vi "WC Get Waveform Subset CDBL.vi"(4 "open interval? (T)":bool=TRUE, 5 "start/duration format":u16(ring) items=["Samples", "Relative Time"], 6 "error in (no error)":errorcluster, 7 "duration":dbl=1.0 format="%0.2f", 8 "start samples/time":dbl format="%0.2f", 9 "Waveform In":cluster{"t0":dbl, "dt":dbl, "Y":cdb[]} {"Y" format="%.3p"; "dt" format="%.6p"; "t0" format="%.6p"}) -> (0 "error out":errorcluster, 1 "actual duration":dbl format="%0.2f", 2 "actual start samples/time":dbl format="%0.2f", 3 "Waveform Out":cluster{"t0":dbl, "dt":dbl, "Y":cdb[]} {"Y" format="%.3p"; "dt" format="%.6p"; "t0" format="%.6p"})   [LabVIEW 2018]
doc: "Retrieves a subset of a waveform at a specified time or index. You must manually select the polymorphic instance you want to use."
panel:
  # "open"
  # "closed"
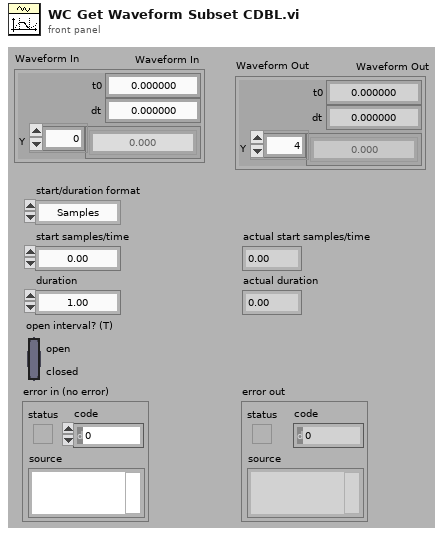
[diagram p1: front panel]
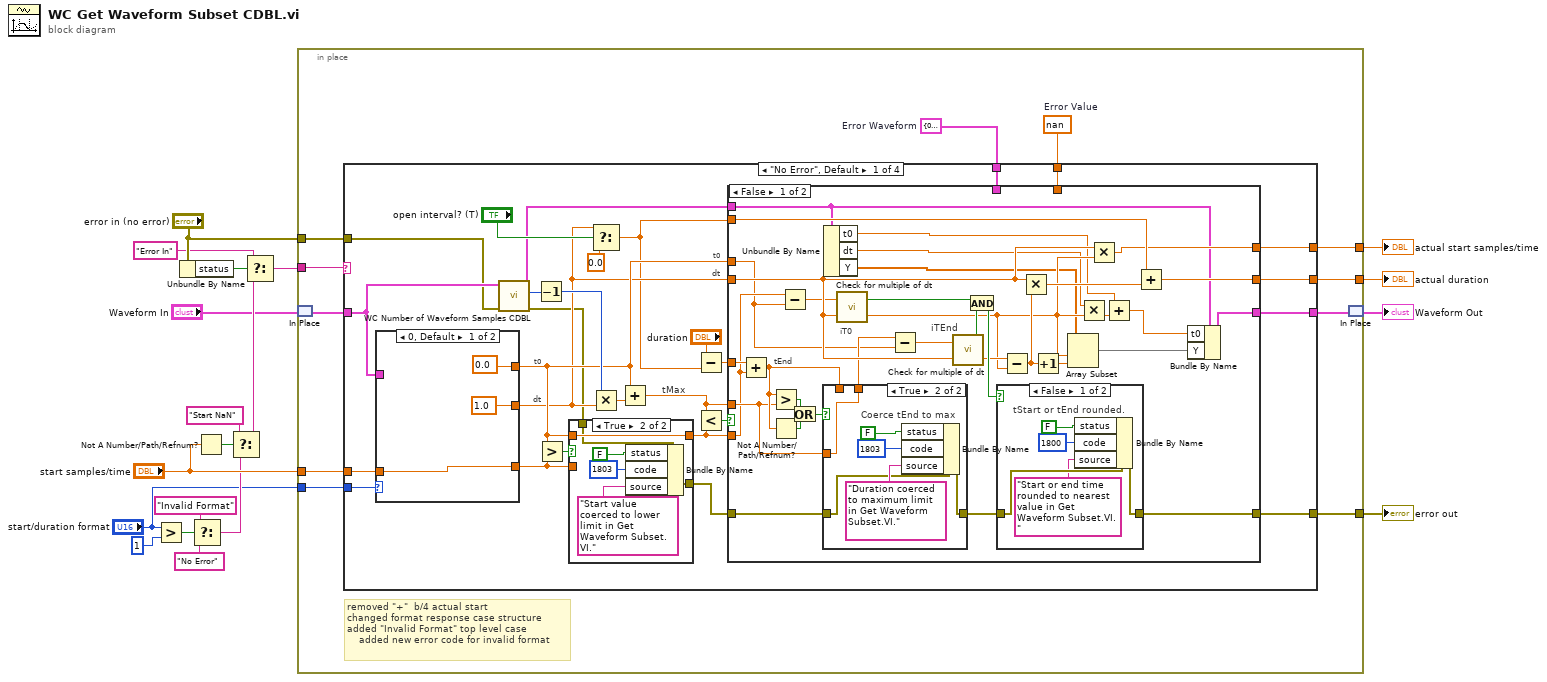
[diagram p0: block diagram]
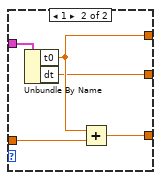
[diagram p2: hidden frame]
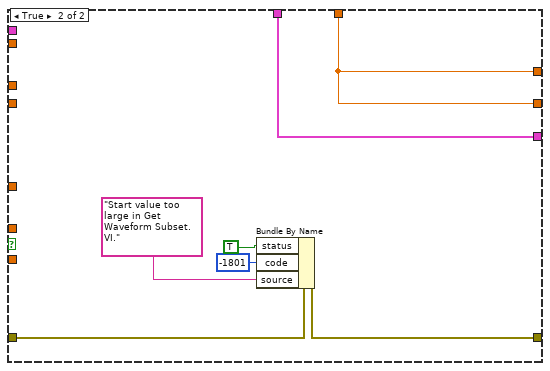
[diagram p5: hidden frame]
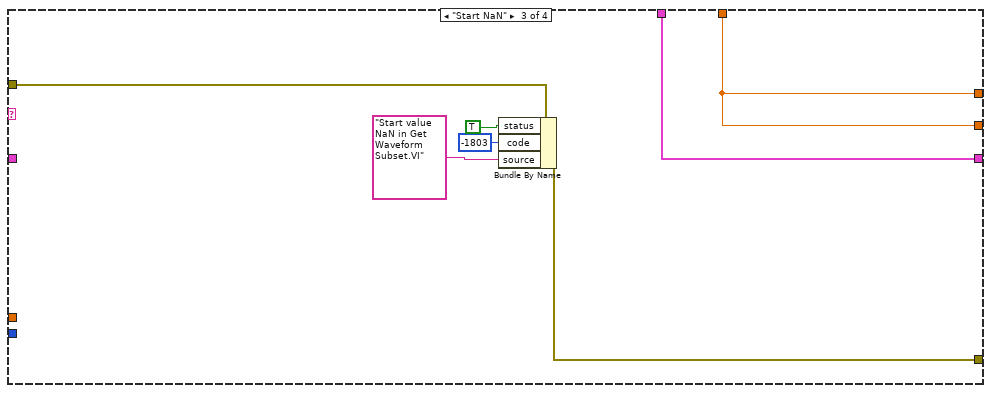
[diagram p8: hidden frame]
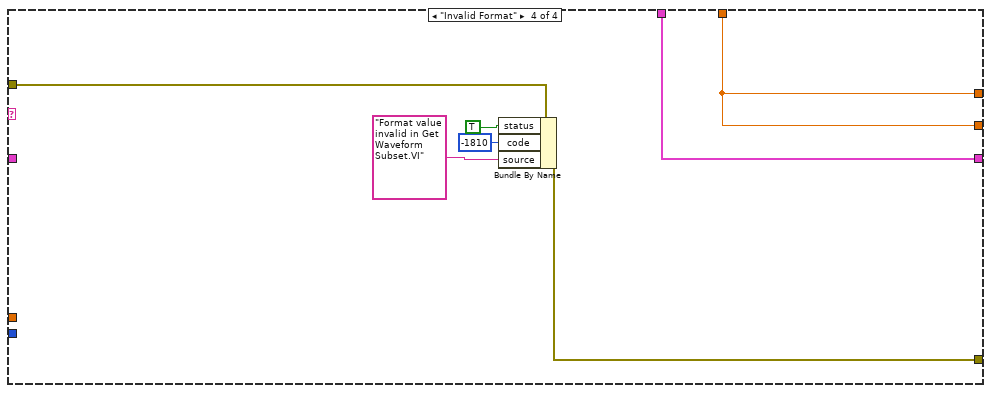
[diagram p9: hidden frame]
diagram:
  n1 = Greater?(x="start/duration format", y=u16 1) -> (0:w7:bool)
  n2 = Unbundle By Name("error in (no error)") -> ("status"=w17:bool)
  n3 = Select(t="Invalid Format", s=w7, f="No Error") -> (s? t:f=w5:string)
  n4 = Not A Number/Path/Refnum?(number/path/refnum="start samples/time") -> (NaN/Path/Refnum?=w19:bool)
  n5 = Select(t="Start NaN", s=w19, f=w5) -> (s? t:f=w15:string)
  n6 = Select(t="Error In", s=w17, f=w15) -> (s? t:f=w12:string)
  n7 = in-place {
    in-place-border: "error in (no error)" -> [w30]
    in-place-border: "start samples/time" -> [w29]
    in-place-border: w12 -> [w28]
    in-place-border: [w27] -> w11
    in-place-border: [w25] -> w10
    in-place-border: [w24] -> w9
    in-place-border: "start/duration format" -> [w23]
    w20 = cluster{"t0":dbl, "dt":dbl, "Y":cdb[]} {"t0"=0.0, "dt"=0.0, "Y"=[]}  # Error Waveform
    w26 = nan  # Error Value
    # "removed \"+\"  b/4 actual start\nchanged format response case structure\nadded \"Invalid Format\" top level case\n    added new error code for invalid format"
    n8 = in-place-match #1("Waveform In") -> (w22:cluster{"t0":dbl, "dt":dbl, "Y":cdb[]})
    n9 = case shown="\"No Error\", Default" w28 {
      tunnel: w22 -> [w33 _ _ _]
      tunnel: w30 -> [w31 w132 w139 w146]
      tunnel: w29 -> [w38 _ _ _]
      tunnel: [w48 w132 w138 w145] -> w27
      tunnel: [w50 w131 w134 w141] -> w21
      tunnel: w20 -> [w49 w131 w134 w141]
      tunnel: [w51 w130 w133 w140] -> w25
      tunnel: w26 -> [w52 w130 w133 w140]
      tunnel: [w47 w130 w133 w140] -> w24
      tunnel: w23 -> [w32 _ _ _]
      frame "No Error", Default {
        # "t0"
        # "dt"
        # "tMax"
        # "t0"
        # "dt"
        n10 = case shown="0, Default" w32 {
          tunnel: [0.0 ("t") w65] -> w45
          tunnel: [1.0 ("t") w64] -> w42
          tunnel: w38 -> [w59 w66]
          tunnel: [w59 w62] -> w37
          tunnel: w33 -> [_ w63]
          frame 0, Default {
          }
          frame 1 {
            n11 = Unbundle By Name(w63) -> ("t0"=w65:dbl, "dt"=w64:dbl)
            n12 = Add(x=w65, y=w66) -> (x+y=w62:dbl)
          }
        }
        n13 = call "WC Number of Waveform Samples CDBL.vi"("error in (no error)"=w31, "Waveform In"=w33) -> ("error out"=w36:errorcluster, "number of samples"=w34:i32, "Waveform Out"=w35:cluster{"t0":dbl, "dt":dbl, "Y":cdb[]})  [unwired: 7 in]
        n14 = Decrement(x=w34) -> (x-1=w58:i32)
        n15 = Greater?(x=w45, y=w37) -> (0:w56:bool)
        n16 = case shown="True" w56 {
          tunnel: w36 -> [w122 w128]
          tunnel: w45 -> [_ w129]
          tunnel: w37 -> [w123 _]
          tunnel: [w123 w129] -> w55
          tunnel: [w122 w127] -> w54
          frame False {
          }
          frame True {
            n17 = Bundle By Name(cluster=w128, "status"=FALSE, "code"=1803, "source"="Start value coerced to lower limit in Get Waveform Subset.VI.") -> (w127:errorcluster)
          }
        }
        n18 = Select(t=w42, s="open interval? (T)", f=0.0) -> (s? t:f=w39:dbl)
        n19 = Multiply(x=w58, y=w42) -> (x*y=w57:dbl)
        n20 = Add(x=w45, y=w57) -> (x+y=w46:dbl)
        n21 = Subtract(x="duration", y=w39) -> (x-y=w41:dbl)
        n22 = Less?(x=w46, y=w55) -> (x < y?=w53:bool)
        n23 = case shown="False" w53 {
          tunnel: w54 -> [w96 w117]
          tunnel: w46 -> [w94 _]
          tunnel: w55 -> [w81 _]
          tunnel: [w90 w121] -> w48
          tunnel: [w76 w116] -> w47
          tunnel: w52 -> [_ w116]
          tunnel: [w74 w116] -> w51
          tunnel: [w67 w115] -> w50
          tunnel: w49 -> [_ w115]
          tunnel: w41 -> [w100 _]
          tunnel: w42 -> [w84 _]
          tunnel: w45 -> [w77 _]
          tunnel: w35 -> [w70 _]
          tunnel: w39 -> [w75 _]
          frame False {
            # "iTEnd"
            # "iT0"
            # "tEnd"
            n24 = Add(x=w100, y=w81) -> (x+y=w95:dbl)
            n25 = Greater?(x=w95, y=w94) -> (0:w99:bool)
            n26 = Not A Number/Path/Refnum?(number/path/refnum=w95) -> (NaN/Path/Refnum?=w98:bool)
            n27 = Subtract(x=w81, y=w77) -> (x-y=w82:dbl)
            n28 = Or(x=w99, y=w98) -> (x .or. y?=w97:bool)
            n29 = case shown="True" w97 {
              tunnel: w96 -> [w108 w111]
              tunnel: [w108 w110] -> w91
              tunnel: w95 -> [w107 _]
              tunnel: w94 -> [_ w109]
              tunnel: [w107 w109] -> w78
              frame False {
                # "tEnd OK,\npass through"
              }
              frame True {
                # "Coerce tEnd to max"
                n30 = Bundle By Name(cluster=w111, "status"=FALSE, "code"=1803, "source"="Duration coerced to maximum limit in Get Waveform Subset.VI.") -> (w110:errorcluster)
              }
            }
            n31 = Unbundle By Name(w70) -> ("t0"=w73:dbl, "dt"=w72:dbl, "Y"=w71:cdb[])
            n32 = call <vilib>:"Check for multiple of dt.vi"("dt"=w84, "time"=w82) -> ("iQuotient"=w83:dbl, "Equal Multiple?"=w92:bool)
            n33 = Subtract(x=w78, y=w77) -> (x-y=w79:dbl)
            n34 = call <vilib>:"Check for multiple of dt.vi"("dt"=w84, "time"=w79) -> ("iQuotient"=w88:dbl, "Equal Multiple?"=w93:bool)
            n35 = And(x=w92, y=w93) -> (x .and. y?=w89:bool)
            n36 = case shown="False" w89 {
              tunnel: w91 -> [w104 w106]
              tunnel: [w105 w106] -> w90
              frame False {
                # "tStart or tEnd rounded."
                n37 = Bundle By Name(cluster=w104, "status"=FALSE, "code"=1800, "source"="Start or end time rounded to nearest value in Get Waveform Subset.VI.") -> (w105:errorcluster)
              }
              frame True {
                # "tStart and tEnd\nnot rounded."
              }
            }
            n38 = Subtract(x=w88, y=w83) -> (x-y=w85:dbl)
            n39 = Multiply(x=w84, y=w85) -> (x*y=w86:dbl)
            n40 = Increment(x=w85) -> (x+1=w87:dbl)
            n41 = Array Subset(array=w71, index=w83, length=w87) -> (w68:cdb[])
            n42 = Multiply(x=w72, y=w83) -> (x*y=w80:dbl)
            n43 = Multiply(x=w84, y=w83) -> (x*y=w74:dbl)
            n44 = Add(x=w73, y=w80) -> (x+y=w69:dbl)
            n45 = Add(x=w75, y=w86) -> (x+y=w76:dbl)
            n46 = Bundle By Name(cluster=w70, "t0"=w69, "Y"=w68) -> (w67:cluster{"t0":dbl, "dt":dbl, "Y":cdb[]})
          }
          frame True {
            n47 = Bundle By Name(cluster=w117, "status"=TRUE, "code"=-1801, "source"="Start value too large in Get Waveform Subset.VI.") -> (w121:errorcluster)
          }
        }
      }
      frame "Error In" {
        # "Incoming Error"
      }
      frame "Start NaN" {
        n48 = Bundle By Name(cluster=w139, "status"=TRUE, "code"=-1803, "source"="Start value NaN in Get Waveform Subset.VI") -> (w138:errorcluster)
      }
      frame "Invalid Format" {
        n49 = Bundle By Name(cluster=w146, "status"=TRUE, "code"=-1810, "source"="Format value invalid in Get Waveform Subset.VI") -> (w145:errorcluster)
      }
    }
    n50 = in-place-match #1(w21) -> (→"Waveform Out":cluster{"t0":dbl, "dt":dbl, "Y":cdb[]})
  }
  "error out" <- w11
  "actual start samples/time" <- w10
  "actual duration" <- w9
